vi "Launch Chart With Slider.vi"   [LabVIEW 2018]
uses:
  <vilib>/ActorFramework/Actor/Actor.lvclass
  modules/mva-core/Source/Mediator/Mediator/Mediator.lvclass
  modules/mva-viewable/Source/IViewable/IViewable Messages/Open Front Panel Msg/Open Front Panel Msg.lvclass
  <vilib>/ActorFramework/Message Enqueuer/Message Priority.ctl
  <vilib>/ActorFramework/Message Enqueuer/Message Enqueuer.lvclass
  modules/mva-viewable/Source/IViewable/IViewable/View Position Enum.ctl
  modules/mva-viewable/Source/IViewable/IViewable/IViewable.lvclass
  ExampleSimpleRootModel/SimpleRootModel.lvclass
  TwoPaneViewManager/TwoPaneViewManager.lvclass
  modules/mva-viewable/Source/IViewManager/IViewManager/IViewManager.lvclass
  SimpleChart/SimpleChart.lvclass
  VerticalSlide/VerticalSlide.lvclass
  SimpleViewModel/SimpleViewModel.lvclass
  78b7b6b9-38c2-4279-a601-2af48d0119de.vi
panel:
  # "This example launches a two-pane MVA application"
types:
  T1 = typedef "MVA Framework.lvlib/IViewable.lvlib/IViewable.lvclass/View Position Enum.ctl" = enum16{"Centered", "Maximized", "Minimized", "Custom", "Unchanged"}
  T2 = typedef "Actor Framework.lvlib/Message Enqueuer.lvclass/Message Priority.ctl" = enum16{"Low", "Normal", "High"}
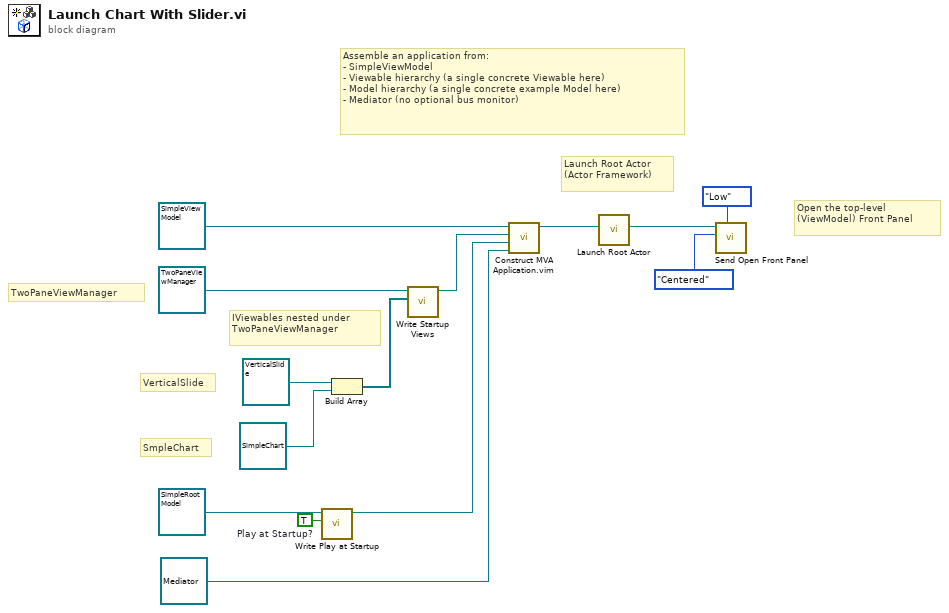
[diagram p0: block diagram]
diagram:
  w2 = TRUE  # Play at Startup?
  # "SmpleChart"
  # "VerticalSlide"
  # "IViewables nested under \nTwoPaneViewManager"
  # "TwoPaneViewManager"
  # "Open the top-level\n(ViewModel) Front Panel"
  # "Launch Root Actor\n(Actor Framework)"
  # "Assemble an application from:\n- SimpleViewModel\n- Viewable hierarchy (a single concrete Viewable here)\n- Model hierarchy (a single concrete example Model here)\n- Mediator (no optional bus monitor)"
  n1 = call "Write Play at Startup.vi"("Play at Startup?"=w2, "SimpleRootModel in"=refnum<class "SimpleRootModel.lvclass"> refnum ("MVAExamples.lvlib:SimpleRootModel.lvclass")) -> ("SimpleRootModel out"=w3:refnum<class "SimpleRootModel.lvclass">)  [unwired: 9 in]
  n2 = Build Array(refnum<class "VerticalSlide.lvclass"> refnum ("MVAExamples.lvlib:VerticalSlide.lvclass"), refnum<class "SimpleChart.lvclass"> refnum ("MVAExamples.lvlib:SimpleChart.lvclass")) -> (w4:refnum<class "IViewable.lvclass">[])
  n3 = call "Write Startup Views.vi"("Startup Views"=w4, "IViewManager in"=refnum<class "TwoPaneViewManager.lvclass"> refnum ("MVAExamples.lvlib:TwoPaneViewManager.lvclass")) -> ("IViewManager out"=w7:refnum<class "TwoPaneViewManager.lvclass">)  [unwired: 9 in]
  n4 = call "Construct MVA Application.vim"("Mediator Type"=refnum<class "Mediator.lvclass"> refnum ("Mediator.lvlib:Mediator.lvclass"), "Model Type"=w3, "Startup View Configuration"=w7, "IViewModel In"=refnum<class "SimpleViewModel.lvclass"> refnum ("MVAExamples.lvlib:SimpleViewModel.lvclass")) -> ("IViewModel Out"=w11:refnum<class "SimpleViewModel.lvclass">)  [unwired: 7 in]
  n5 = call <vilib>:"Launch Root Actor.vi"("Actor"=w11) -> ("Actor's Enqueuer"=w10:refnum<class "Message Enqueuer.lvclass">)  [unwired: 9 in, 1 out]
  n6 = call "Send Open Front Panel.vi"("Message Priority (Normal)"=Message_Priority."Low", "Position"=View_Position_Enum."Centered", "Message Enqueuer"=w10) -> ()  [unwired: 7 in, 2 out]
